vi "start.vi"(8 "error in (no error)":errorcluster, 11 "queue_size":i32=10) -> (0 "error out":errorcluster)   [LabVIEW 2015, in "lv-recipe-machine.lvlib"]
doc: "start.vi can be used to start the business logic of the recipe_machine. It will output the references to interact with the recipe_machine module."
uses:
  lv-recipe-machine.lvlib
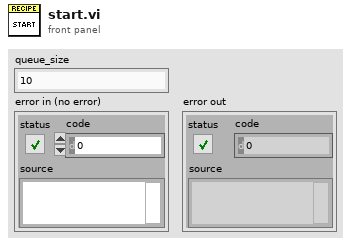
[diagram p1: front panel]
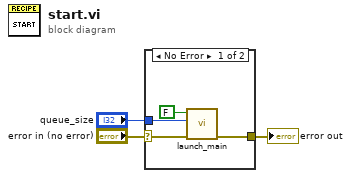
[diagram p0: block diagram]
diagram:
  n1 = case shown="No Error" "error in (no error)" {
    selector: "error in (no error)" -> [w5 w8]
    tunnel: [w7 w8] -> w2
    tunnel: "queue_size" -> [w4 _]
    frame No Error {
      n2 = call "launch_main.vi"("error in (no error)"=w5, "queue_size"=w4, "run_f_stop_t"=FALSE ("Run(F)/Abort(T)")) -> ("error out"=w7:errorcluster)  [unwired: 8 in]
    }
    frame Error {
    }
  }
  "error out" <- w2
